vi "PowerLineConf.vi"(6 "Power Line\nEnable":bool=TRUE, 8 "Power Line":T2, 9 "Power Line\nChannel":tag="PXIe-4309/ai0") -> (3 "Power Line\nConfiguration":T1={"Line Name"="", "Physical Channel"="PXIe-4309/ai0", "Shunt Resistor [Ohm]"=0.0, "Min Current [A]"=0.0, "Max Current [A]"=0.0, "Enable"=FALSE} {"Max Current [A]" format="%#_13g"; "Min Current [A]" format="%#_13g"; "Shunt Resistor [Ohm]" format="%#_13g"})   [LabVIEW 2020]
uses:
  HiFiveUnmatchedPowerLine.ctl
  HiFiveUnmatchedPowerLineConfig.ctl
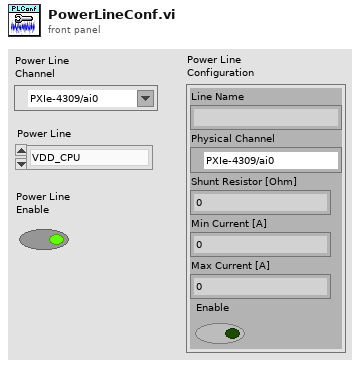
[diagram p1: front panel]
types:
  T1 = typedef "HiFiveUnmatchedPowerLineConfig.ctl" = cluster{"Line Name":string, "Physical Channel":tag, "Shunt Resistor [Ohm]":dbl, "Min Current [A]":dbl, "Max Current [A]":dbl, "Enable":bool}
  T2 = typedef "HiFiveUnmatchedPowerLine.ctl" = enum8{"VDD_CPU", "VDD_DDR_SOC", "VDD_IO", "VDD_PLL", "VDD_PCIEVP", "VDD_PCIEVPH", "VDD_DDR_MEM", "VDD_DDRPLL", "VDD_DDRVPP"}
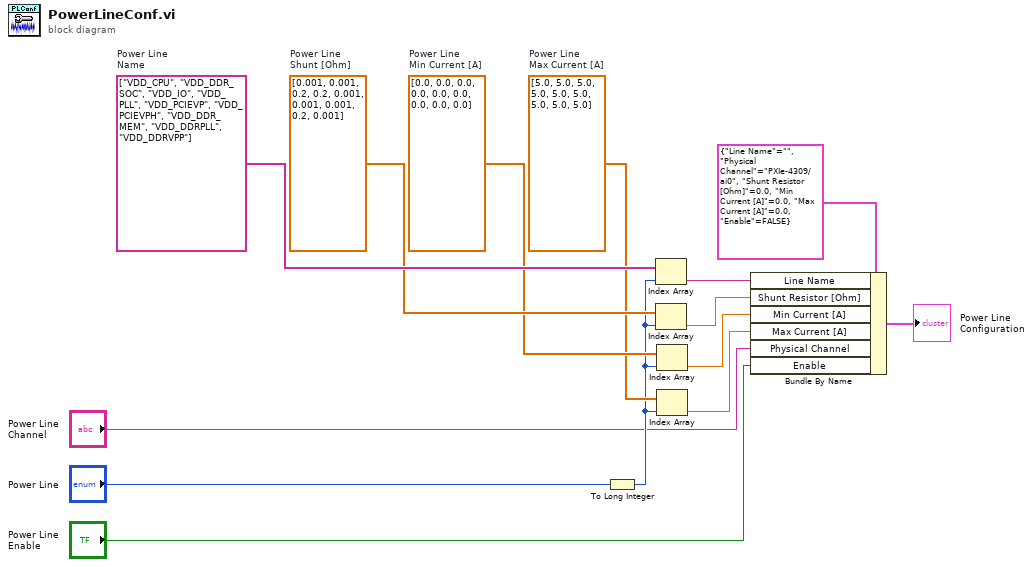
[diagram p0: block diagram]
diagram:
  w8 = dbl[] [5.0, 5.0, 5.0, 5.0, 5.0, 5.0, 5.0, 5.0, 5.0]  # Power Line Max Current [A]
  w9 = dbl[] [0.0, 0.0, 0.0, 0.0, 0.0, 0.0, 0.0, 0.0, 0.0]  # Power Line Min Current [A]
  w10 = dbl[] [0.001, 0.001, 0.2, 0.2, 0.001, 0.001, 0.001, 0.2, 0.001]  # Power Line Shunt [Ohm]
  w11 = string[] ["VDD_CPU", "VDD_DDR_SOC", "VDD_IO", "VDD_PLL", "VDD_PCIEVP", "VDD_PCIEVPH", "VDD_DDR_MEM", "VDD_DDRPLL", "VDD_DDRVPP"]  # Power Line Name
  n1 = To Long Integer(number="Power Line") -> (32bit integer=w7:i32)
  n2 = Index Array(array=w11, index=w7) -> (element=w6:string)
  n3 = Index Array(array=w10, index=w7) -> (element=w5:dbl)
  n4 = Index Array(array=w9, index=w7) -> (element=w4:dbl)
  n5 = Index Array(array=w8, index=w7) -> (element=w3:dbl)
  n6 = Bundle By Name(cluster=T1 {"Line Name"="", "Physical Channel"="PXIe-4309/ai0", "Shunt Resistor [Ohm]"=0.0, "Min Current [A]"=0.0, "Max Current [A]"=0.0, "Enable"=FALSE} ("HiFive Unmatched\nPower Monitor Line Configuration"), "Line Name"=w6, "Shunt Resistor [Ohm]"=w5, "Min Current [A]"=w4, "Max Current [A]"=w3, "Physical Channel"="Power Line\nChannel", "Enable"="Power Line\nEnable") -> (→"Power Line\nConfiguration":T1)
